vi "RobotDll (SubVI).vi"(0 "rcm xyz command":cluster{"x":dbl, "y":dbl, "z":dbl}, 1 "ArmPower":bool, 2 "Control Mode":bool, 3 "XYZ Stage Power":bool, 4 "E-STOP button":bool caption="Stop Button", 5 "robot xyz command":T2, 6 "ArmID":i32, 7 "Run":bool, 10 "Stop Button in":bool caption="Stop Button", 11 "joint command":T1) -> (12 "rcm":cluster{"x":dbl, "y":dbl, "z":dbl}, 13 "Stop Button out":bool, 14 "Tooltip":T2, 15 "ReceiveCount":u64, 17 "ActualJointAngles":T1, 18 "SendCount":u64, 19 "RobotConnection":bool)   [LabVIEW 2016]
uses:
  EyeRobotDLL.dll
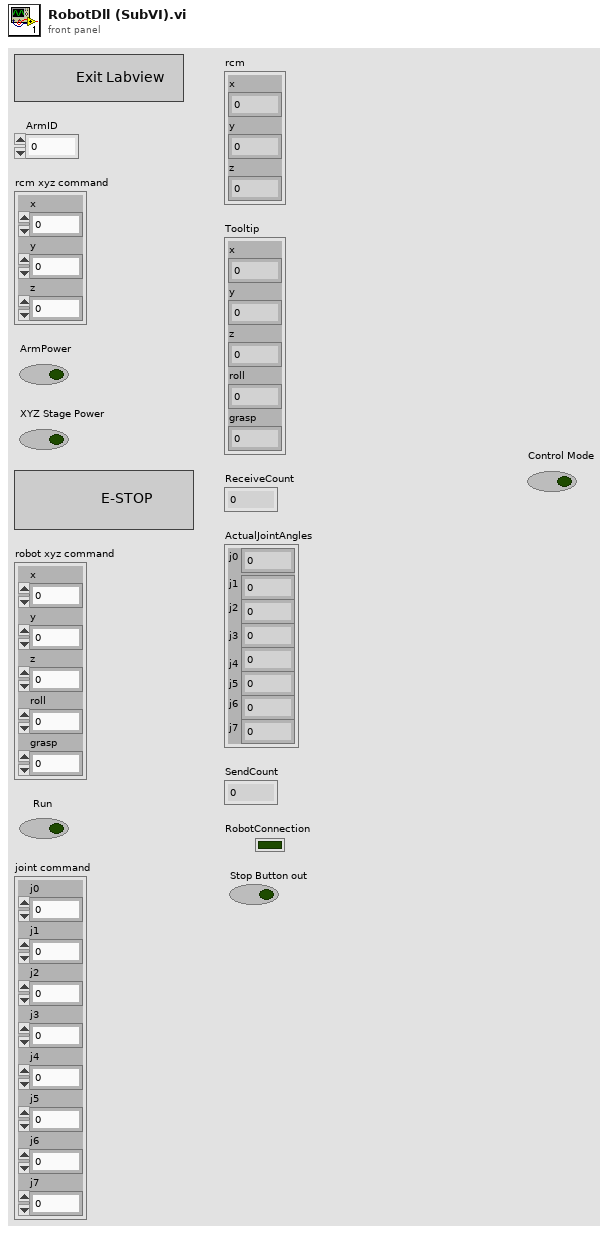
[diagram p1: front panel]
types:
  T1 = cluster{"j0":dbl, "j1":dbl, "j2":dbl, "j3":dbl, "j4":dbl, "j5":dbl, "j6":dbl, "j7":dbl}
  T2 = cluster{"x":dbl, "y":dbl, "z":dbl, "roll":dbl, "grasp":dbl}
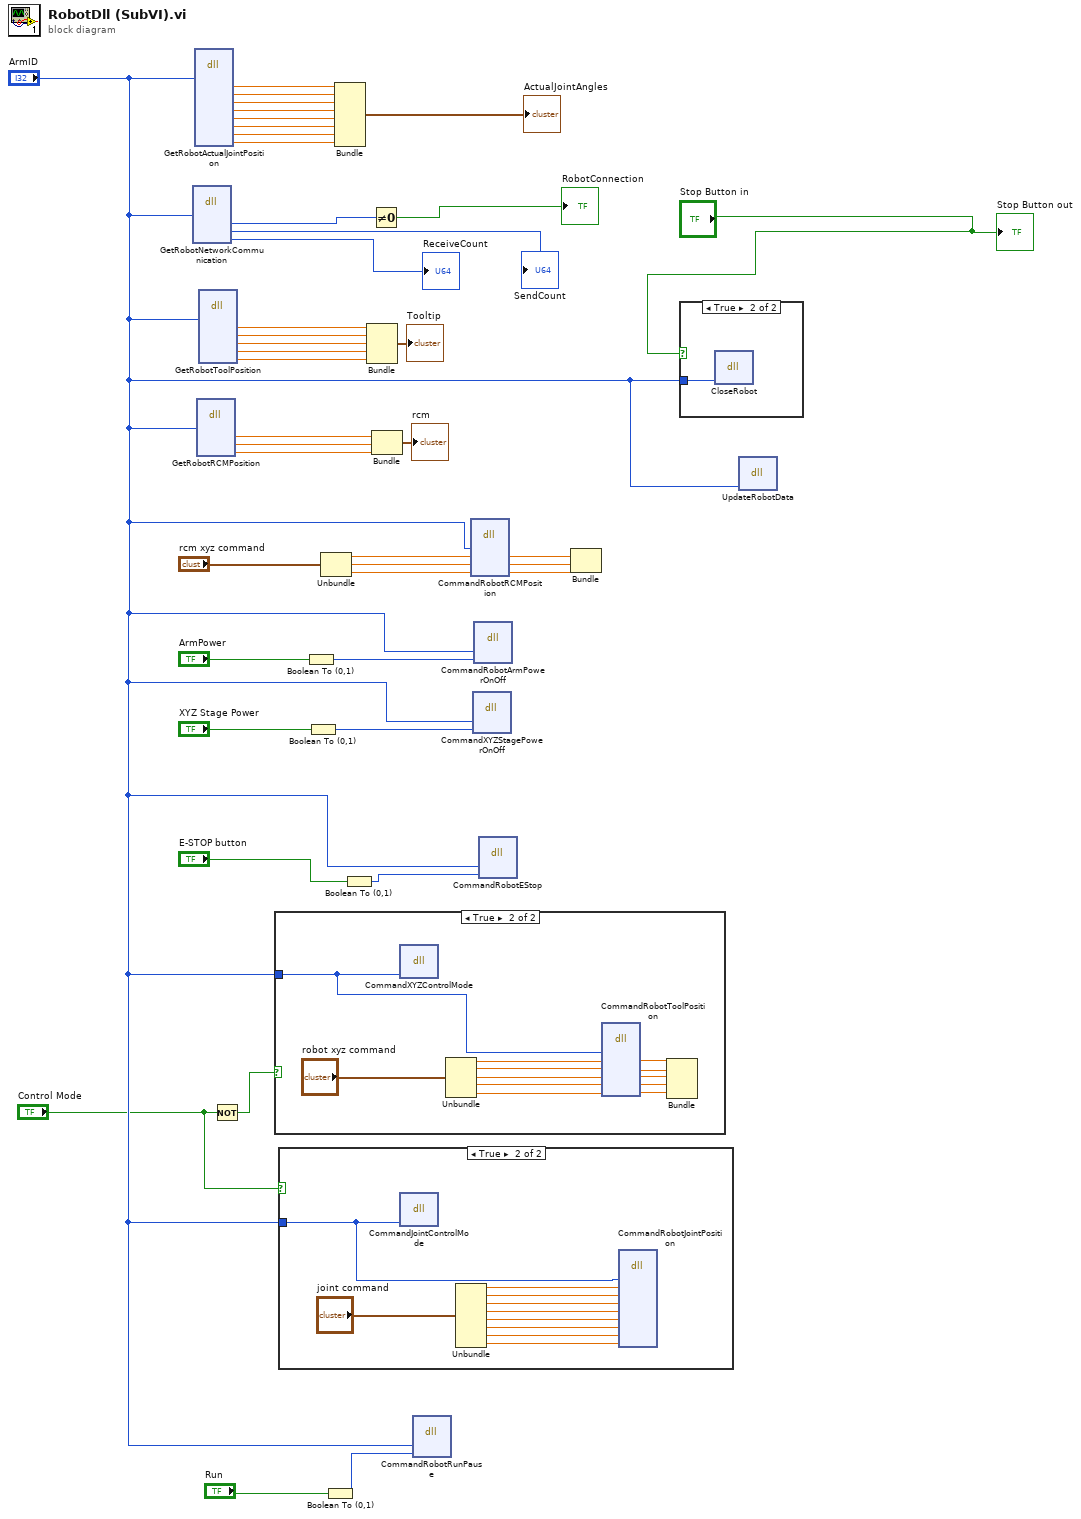
[diagram p0: block diagram]
diagram:
  n1 = dll-call lib="D:/Kevin/IRISS V2 dev/Host Demo/Functions/EyeRobotDLL.dll" fn="GetRobotNetworkCommunication"("id"="ArmID") -> ("RobotConnected"=w16:i32, "SendCount"=→"SendCount":u64, "ReceiveCount"=→"ReceiveCount":u64)  [unwired: 8 in, 2 out]
  n2 = dll-call lib="D:/Kevin/IRISS V2 dev/Host Demo/Functions/EyeRobotDLL.dll" fn="GetRobotActualJointPosition"("armID"="ArmID") -> ("j0"=w18:dbl, "j1"=w19:dbl, "j2"=w20:dbl, "j3"=w21:dbl, "j4"=w22:dbl, "j5"=w23:dbl, "j6"=w24:dbl, "j7"=w25:dbl)  [unwired: 13 in, 2 out]
  n3 = dll-call lib="D:/Kevin/IRISS V2 dev/Host Demo/Functions/EyeRobotDLL.dll" fn="GetRobotRCMPosition"("id"="ArmID") -> ("x"=w33:dbl, "y"=w34:dbl, "z"=w35:dbl)  [unwired: 8 in, 2 out]
  n4 = dll-call lib="D:/Kevin/IRISS V2 dev/Host Demo/Functions/EyeRobotDLL.dll" fn="GetRobotToolPosition"("id"="ArmID") -> ("x"=w27:dbl, "y"=w28:dbl, "z"=w29:dbl, "roll"=w30:dbl, "grasp"=w31:dbl)  [unwired: 10 in, 2 out]
  n5 = Not(x="Control Mode") -> (.not. x?=w5:bool)
  n6 = case shown="True" w5 {
    tunnel: "ArmID" -> [_ w43]
    frame False {
    }
    frame True {
      n7 = dll-call lib="D:/Kevin/IRISS V2 dev/Host Demo/Functions/EyeRobotDLL.dll" fn="CommandXYZControlMode"("id"=w43) -> ()  [unwired: 5 in, 2 out]
      n8 = Unbundle("robot xyz command") -> ("x"=w48:dbl, "y"=w47:dbl, "z"=w46:dbl, "roll"=w45:dbl, "grasp"=w44:dbl)
      n9 = dll-call lib="D:/Kevin/IRISS V2 dev/Host Demo/Functions/EyeRobotDLL.dll" fn="CommandRobotToolPosition"("id"=w43, "x"=w48, "y"=w47, "z"=w46, "roll"=w45, "grasp"=w44) -> ("x"=w54:dbl, "y"=w53:dbl, "z"=w52:dbl, "roll"=w51:dbl, "grasp"=w50:dbl)  [unwired: 5 in, 2 out]
      n10 = Bundle("x"=w54, "y"=w53, "z"=w52, "roll"=w51, "grasp"=w50) -> ()  [unwired: 1 in, 1 out]
    }
  }
  n11 = case shown="True" "Control Mode" {
    tunnel: "ArmID" -> [_ w55]
    frame False {
    }
    frame True {
      n12 = dll-call lib="D:/Kevin/IRISS V2 dev/Host Demo/Functions/EyeRobotDLL.dll" fn="CommandJointControlMode"("id"=w55) -> ()  [unwired: 5 in, 2 out]
      n13 = Unbundle("joint command") -> ("j0"=w63:dbl, "j1"=w62:dbl, "j2"=w61:dbl, "j3"=w60:dbl, "j4"=w59:dbl, "j5"=w58:dbl, "j6"=w57:dbl, "j7"=w56:dbl)
      n14 = dll-call lib="D:/Kevin/IRISS V2 dev/Host Demo/Functions/EyeRobotDLL.dll" fn="CommandRobotJointPosition"("id"=w55, "j0"=w63, "j1"=w62, "j2"=w61, "j3"=w60, "j4"=w59, "j5"=w58, "j6"=w57, "j7"=w56) -> ()  [unwired: 13 in, 2 out]
    }
  }
  n15 = Boolean To (0,1)(Boolean="ArmPower") -> (0, 1=w1:i16)
  n16 = Boolean To (0,1)(Boolean="XYZ Stage Power") -> (0, 1=w4:i16)
  n17 = Unbundle("rcm xyz command") -> ("x"=w10:dbl, "y"=w11:dbl, "z"=w12:dbl)
  n18 = Boolean To (0,1)(Boolean="Run") -> (0, 1=w37:i16)
  n19 = Bundle("j0"=w18, "j1"=w19, "j2"=w20, "j3"=w21, "j4"=w22, "j5"=w23, "j6"=w24, "j7"=w25) -> (→"ActualJointAngles":T1)  [unwired: 1 in]
  n20 = Boolean To (0,1)(Boolean="E-STOP button") -> (0, 1=w41:i16)
  n21 = Bundle("x"=w27, "y"=w28, "z"=w29, "roll"=w30, "grasp"=w31) -> (→"Tooltip":T2)  [unwired: 1 in]
  n22 = Not Equal To 0?(x=w16) -> (x != 0?=→"RobotConnection":bool)
  n23 = Bundle("x"=w33, "y"=w34, "z"=w35) -> (→"rcm":cluster{"x":dbl, "y":dbl, "z":dbl})  [unwired: 1 in]
  n24 = dll-call lib="D:/Kevin/IRISS V2 dev/Host Demo/Functions/EyeRobotDLL.dll" fn="CommandRobotRunPause"("id"="ArmID", "RunPause"=w37) -> ()  [unwired: 6 in, 2 out]
  n25 = dll-call lib="D:/Kevin/IRISS V2 dev/Host Demo/Functions/EyeRobotDLL.dll" fn="CommandRobotRCMPosition"("id"="ArmID", "x"=w10, "y"=w11, "z"=w12) -> ("x"=w6:dbl, "y"=w7:dbl, "z"=w8:dbl)  [unwired: 5 in, 2 out]
  n26 = dll-call lib="D:/Kevin/IRISS V2 dev/Host Demo/Functions/EyeRobotDLL.dll" fn="CommandXYZStagePowerOnOff"("id"="ArmID", "OnOff"=w4) -> ()  [unwired: 6 in, 2 out]
  n27 = dll-call lib="D:/Kevin/IRISS V2 dev/Host Demo/Functions/EyeRobotDLL.dll" fn="CommandRobotArmPowerOnOff"("id"="ArmID", "OnOff"=w1) -> ()  [unwired: 6 in, 2 out]
  n28 = dll-call lib="D:/Kevin/IRISS V2 dev/Host Demo/Functions/EyeRobotDLL.dll" fn="CommandRobotEStop"("id"="ArmID", "estop"=w41) -> ()  [unwired: 6 in, 2 out]
  n29 = Bundle("x"=w6, "y"=w7, "z"=w8) -> ()  [unwired: 1 in, 1 out]
  n30 = case shown="True" "Stop Button in" {
    tunnel: "ArmID" -> [_ w65]
    frame False {
    }
    frame True {
      n31 = dll-call lib="D:/Kevin/IRISS V2 dev/Host Demo/Functions/EyeRobotDLL.dll" fn="CloseRobot" label="Close"("id"=w65) -> ()  [unwired: 5 in, 2 out]
    }
  }
  n32 = dll-call lib="D:/Kevin/IRISS V2 dev/Host Demo/Functions/EyeRobotDLL.dll" fn="UpdateRobotData"("id"="ArmID") -> ()  [unwired: 5 in, 2 out]
  "Stop Button out" <- "Stop Button in"
